vi "myRIO_CriticalMainTest.vi"() -> ()   [LabVIEW 2014]
panel:
  in  "Stop":bool
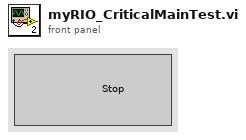
[diagram p1: front panel]
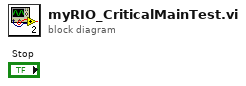
[diagram p0: block diagram]
diagram:
